vi "XYStage.MoveAbsolute(real).vi"(8 "error in (no error)":errorcluster, 10 "Position":T2, 11 "XYStage":refnum<class "XYStage.lvclass">) -> (0 "error out":errorcluster, 2 "Absolute counts":T1, 3 "XYStage out":refnum<class "XYStage.lvclass">)   [LabVIEW 2013, in "XYStage.lvclass"]
doc: "---------------------------------------------------------------\nJKI State Machine Objects™\nhttp://jki.net/state-machine-objects/\nCopyright (C) 2005-2015, JKI <info@jki.net>\nALL RIGHTS RESERVEDJKI State Machine Objects (SMO) 1.0.0.5\nJKI - JKI\nCopyright (c) 2016, JKI"
uses:
  XYStage.lvclass
  Typedefs/(real)Coords--Cluster.ctl
  Typedefs/(counts)Coords--Cluster.ctl
panel:
  # "For instructions on how to use the JKI State Machine Objects, examples and video tutorials, visit:\nhttp://jki.net/state-machine-objects/\n\nJKI State Machine Objects™\nhttp://jki.net/state-machine-objects/\nCopyright (C) 2005-2015, JKI <info@jki.net>\nALL RIGHTS RESERVED"
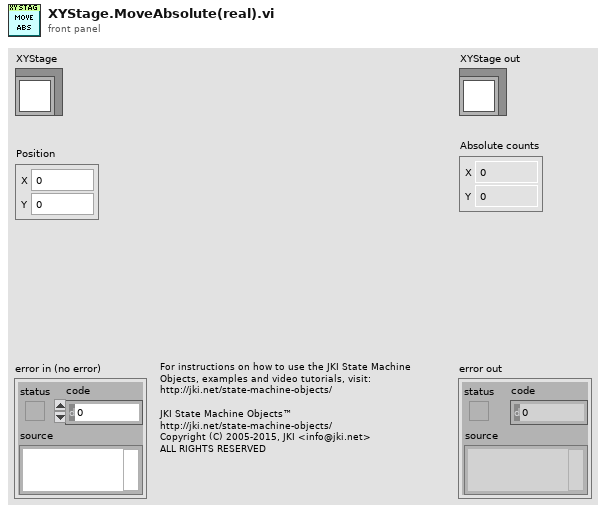
[diagram p1: front panel]
types:
  T1 = typedef "XYStage.lvclass/(counts)Coords--Cluster.ctl" = cluster{"X":i32, "Y":i32}
  T2 = typedef "XYStage.lvclass/(real)Coords--Cluster.ctl" = cluster{"X":dbl, "Y":dbl}
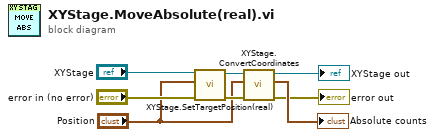
[diagram p0: block diagram]
diagram:
  n1 = call "XYStage.SetTargetPosition(real).vi"("error in (no error)"="error in (no error)", "Target Position"="Position", "XYStage"="XYStage") -> ("error out"=w3:errorcluster, "XYStage out"=w5:refnum<class "XYStage.lvclass">)  [unwired: 6 in, 1 out]
  n2 = call-dynamic "XYStage.ConvertCoordinates.vi"("error in (no error)"=w3, "Real Units Coords"="Position", "XYStage in"=w5) -> ("error out"=→"error out":errorcluster, "Counts out"=→"Absolute counts":T1, "XYStage out"=→"XYStage out":refnum<class "XYStage.lvclass">)  [unwired: 5 in, 1 out]
